vi "Format Read Command.vi"(4 "error in":errorcluster, 5 "Variable to Read":T1, 6 "Flow Meter DevID":i32=1, 7 "VISA resource name":refnum<visa-resource-name>) -> (0 "error out":errorcluster, 1 "Length Bytes (Dec)":i32, 2 "Command String with Checksum":string, 3 "VISA resource name out":refnum<visa-resource-name>)   [LabVIEW 2012, in "FEM-03.lvlib"]
uses:
  FEM-03.lvlib
  Controls/Variable List.ctl
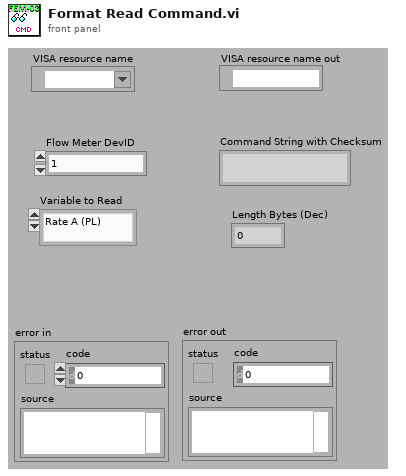
[diagram p1: front panel]
types:
  T1 = typedef "FEM-03.lvlib/Variable List.ctl" = enum16{"Rate A (PL)", "Rate A (GT)", "Job Total A", "Grand Total A", "A-KFR for Rate", "A-KFR decimal point location", "A-KFT for Total", "A-KFT decimal point location ", "A-Rate Engineering Units", "A-Total Engineering units", "A-Flow Direction", "Rate B (PL)", "Rate B (GT)", "Job Total B", "Grand Total B", "B-KFR for Rate", "B-KFR deciminal point location", "B-Rate Engineering units", "B-KFT for Total", "B-KFT decimal point location", "B-Total Engineering units", "Limit 1 Mode", "Limit1", "Margin 1 for rate limit", "Limit 2 Mode", "Limit2", "Margin 2 for rate limit", "Milli-amps Offset", "Milli-amps Out", "Analog Out Mode", "Serial Speed", "Unit Number", "Serial RESET TOTAL", "Update EEPROM", "Relay Override", "FORCE mA Output"}
  T2 = typedef "FEM-03.lvlib/Variable Info.ctl" = cluster{"Hex Address (String)":string, "Length Bytes (String)":string, "Length Bytes (Dec)":i32, "Multibyte format":enum16{"MSB First", "Array last digit 0", "None"}}
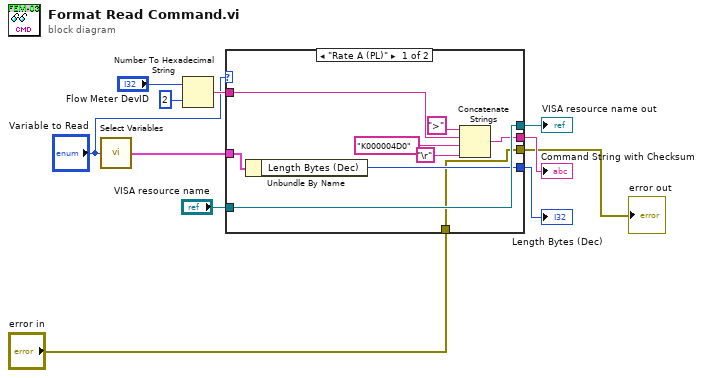
[diagram p0: block diagram]
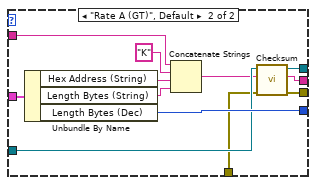
[diagram p2: hidden frame]
diagram:
  n1 = call "Select Variables.vi"("Variables"="Variable to Read") -> ("Variable Info"=w8:T2)
  n2 = Number To Hexadecimal String(1:i16 2 ("width (-)"), 2:"Flow Meter DevID") -> (0:w7:string)
  n3 = case shown="\"Rate A (PL)\"" "Variable to Read" {
    tunnel: [w14 w32] -> w11
    tunnel: "VISA resource name" -> [w20 w31]
    tunnel: [w20 w30] -> w9
    tunnel: w8 -> [w15 w28]
    tunnel: w7 -> [w19 w24]
    tunnel: [w16 w23] -> w4
    tunnel: [w13 w22] -> w2
    tunnel: "error in" -> [w13 w21]
    frame "Rate A (PL)" {
      n4 = Unbundle By Name(w15) -> ("Length Bytes (Dec)"=w14:i32)
      n5 = Concatenate Strings(">" ("string"), w19, "K000004D0" ("Command String with Checksum"), "\r") -> (w16:string)
    }
    frame "Rate A (GT)", Default {
      n6 = Unbundle By Name(w28) -> ("Hex Address (String)"=w26:string, "Length Bytes (String)"=w27:string, "Length Bytes (Dec)"=w32:i32)
      n7 = Concatenate Strings(w24, "K" ("string"), w26, w27) -> (w29:string)
      n8 = call "Checksum.vi"("error in"=w21, "Command String"=w29, "VISA resource name"=w31) -> ("error out"=w22:errorcluster, "Command String with Checksum"=w23:string, "VISA resource name out"=w30:refnum<visa-resource-name>)  [unwired: 5 in, 1 out]
    }
  }
  "Length Bytes (Dec)" <- w11
  "Command String with Checksum" <- w4
  "VISA resource name out" <- w9
  "error out" <- w2
